vi "WinBuilder._2vi.vi"(6 "nSampleNeeded":i32, 7 "TimeStampNeeded":ext, 8 "Error In":errorcluster, 10 "Wvfrm_ref":T2={"t0"=timestamp(0 s since 1904-01-01), "dt"=1.0, "attributes"=variant, "Y_ref"=refnum} {"dt" format="%0.6f"; "t0" format="%<%X\n%x>T"}, 11 "Fitter In":refnum<class "FitterBase.lvclass">) -> (0 "Error Out":errorcluster, 1 "Valid":bool, 2 "Window":T1={"Timestamp"=0.0, "Samples"=[], "Window Valid"=FALSE, "T0"=-1.0} {"T0" format="%.6f"; "Timestamp" format="%.6f"}, 3 "Fitter Out":refnum<class "FitterBase.lvclass">, 4 "Continue":bool)   [LabVIEW 2018, in "AnalysisPlugins.lvlib" / "FitterBase.lvclass"]
uses:
  FitterBase.lvclass
  Typedefs/clAnalysisConfig.ctl
  Digitizer/DigitizerPlugins/DigitizerBaseClass/Typedefs/WfrmAttributes.ctl
  Digitizer/DigitizerPlugins/DigitizerBaseClass/DigitizerBase.lvclass
  Typedefs/Wvfrm_ref.ctl
  AnalysisPluginBaseClass/Typedefs/clWindowData.ctl
  AnalysisPluginBaseClass/AnalysisPluginsBase.lvclass
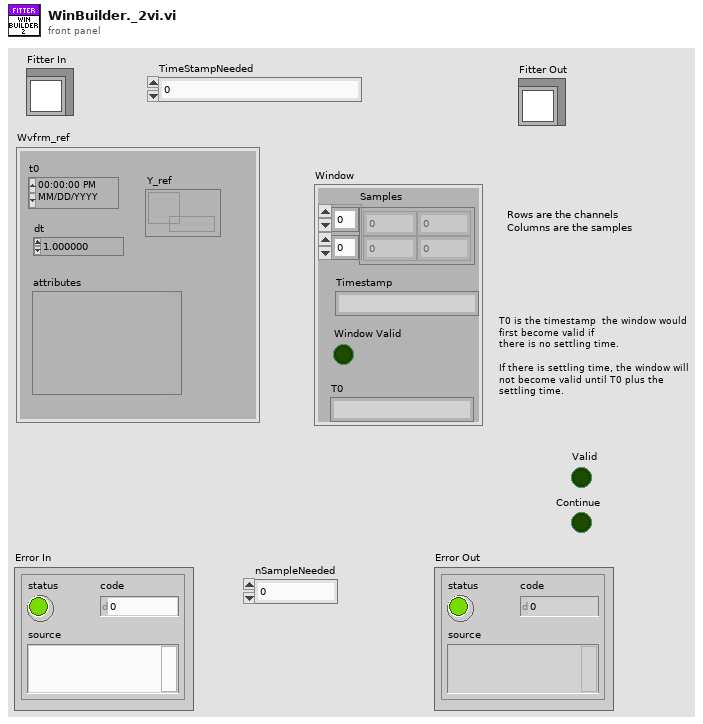
[diagram p1: front panel]
types:
  T1 = typedef "AnalysisPlugins.lvlib/AnalysisPluginsBase.lvclass/clWindowData.ctl" = cluster{"Timestamp":ext, "Samples":dbl[][], "Window Valid":bool, "T0":ext}
  T2 = typedef "AnalysisPlugins.lvlib/FitterBase.lvclass/Wvfrm_ref.ctl" = cluster{"t0":timestamp, "dt":dbl, "attributes":variant, "Y_ref":refnum<data-value>}
  T3 = typedef "DigitizerPlugins.lvlib/DigitizerBase.lvclass/WfrmAttributes.ctl" = cluster{"XOffset":dbl, "ActualPts":i64, "FirstValid":i64}
  T4 = typedef "AnalysisPlugins.lvlib/FitterBase.lvclass/clAnalysisConfig.ctl" = cluster{"F0":u32, "SettlingTime":dbl, "AnalysisCycles":dbl, "SampleRate":dbl, "NumChannels":u32, "TsOffset":enum16{"start", "middle", "end"}}
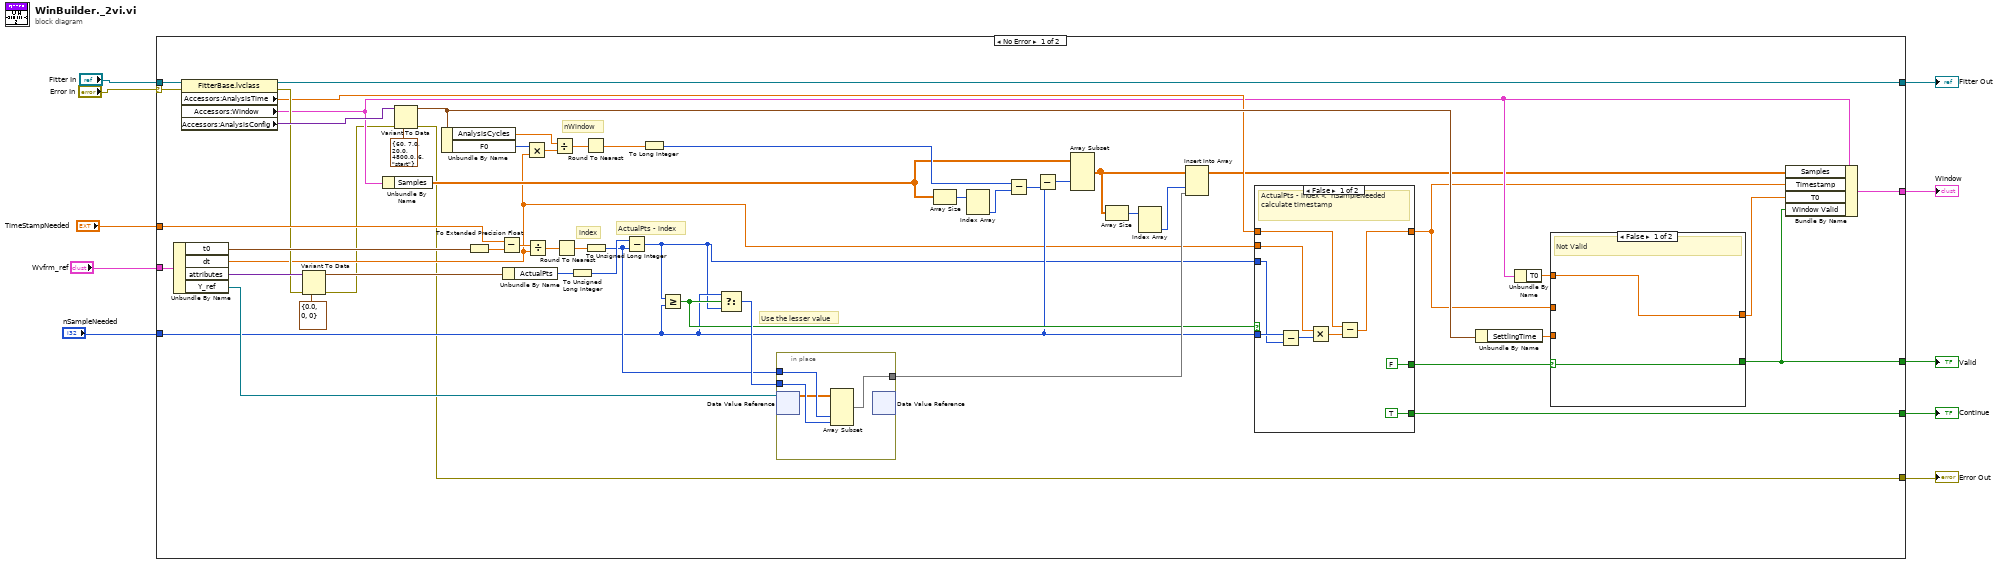
[diagram p0: block diagram]
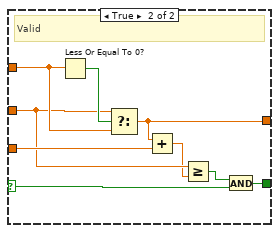
[diagram p2: hidden frame]
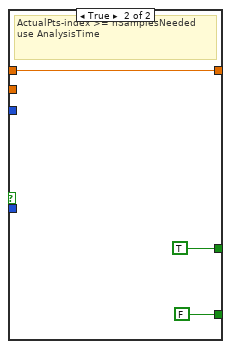
[diagram p3: hidden frame]
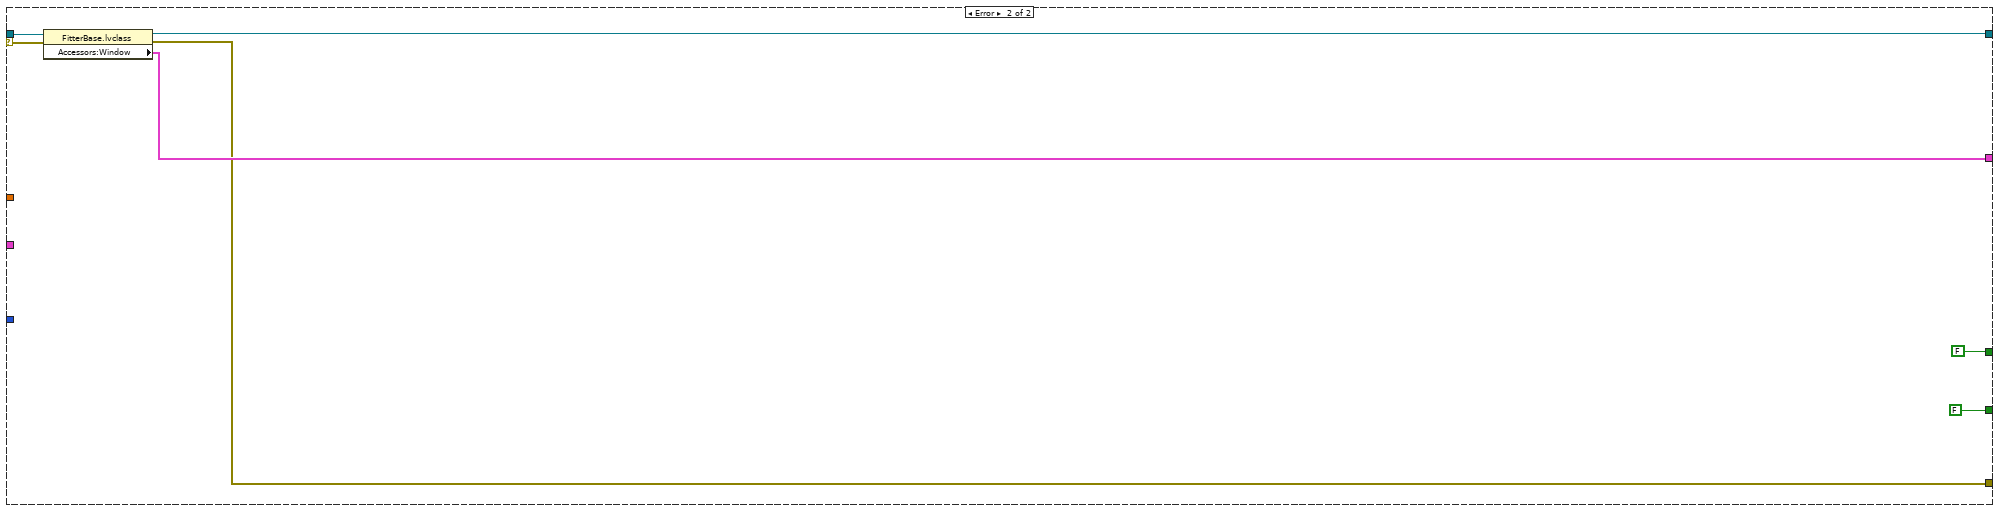
[diagram p4: hidden frame]
diagram:
  n1 = case shown="No Error" "Error In" {
    selector: "Error In" -> [w63 w97]
    tunnel: "Fitter In" -> [w64 w98]
    tunnel: "Wvfrm_ref" -> [w60 _]
    tunnel: "TimeStampNeeded" -> [w57 _]
    tunnel: "nSampleNeeded" -> [w27 _]
    tunnel: [w23 FALSE] -> w5
    tunnel: [w15 FALSE] -> w4
    tunnel: [w14 w94] -> w3
    tunnel: [w13 w93] -> w2
    tunnel: [w11 w92] -> w1
    frame No Error {
      # "nWindow"
      # "Use the lesser value"
      # "ActualPts - index"
      # "index"
      n2 = Unbundle By Name(w60) -> ("t0"=w59:timestamp, "dt"=w25:dbl, "attributes"=w54:variant, "Y_ref"=w47:refnum<data-value>)
      n3 = property class="FitterBase.lvclass"(reference=w64, error in=w63) -> (reference out=w13:refnum<class "FitterBase.lvclass">, error out=w52:errorcluster, "Accessors:AnalysisTime"=w24:dbl, "Accessors:Window"=w22:T1, "Accessors:AnalysisConfig"=w62:variant)
      n4 = Variant To Data(error in=w52, type=T3 {"XOffset"=0.0, "ActualPts"=0, "FirstValid"=0} ("Attributes"), Variant=w54) -> (data=w51:T3, error out=w12:errorcluster)
      n5 = Unbundle By Name(w22) -> ("Samples"=w36:dbl[][])
      n6 = Variant To Data(error in=w12, type=T4 {"F0"=60, "SettlingTime"=7.0, "AnalysisCycles"=20.0, "SampleRate"=4800.0, "NumChannels"=6, "TsOffset"=enum."start"} ("clAnalysisConfig"), Variant=w62) -> (data=w43:T4, error out=w11:errorcluster)
      n7 = Unbundle By Name(w43) -> ("AnalysisCycles"=w40:dbl, "F0"=w42:u32)
      n8 = To Extended Precision Float(1:w59) -> (0:w58:ext)
      n9 = Subtract(x=w57, y=w58) -> (x-y=w56:ext)
      n10 = Unbundle By Name(w51) -> ("ActualPts"=w49:i64)
      n11 = Multiply(x=w42, y=w25) -> (x*y=w41:dbl)
      n12 = Divide(x=w56, y=w25) -> (x/y=w55:ext)
      n13 = Divide(x=w40, y=w41) -> (x/y=w39:dbl)
      n14 = Round To Nearest(number=w55) -> (nearest integer value=w50:ext)
      n15 = To Unsigned Long Integer(number=w49) -> (unsigned 32bit integer=w48:u32)
      n16 = Round To Nearest(number=w39) -> (nearest integer value=w38:dbl)
      n17 = To Unsigned Long Integer(number=w50) -> (unsigned 32bit integer=w45:u32)
      n18 = Subtract(x=w48, y=w45) -> (x-y=w26:u32)
      n19 = To Long Integer(number=w38) -> (32bit integer=w37:i32)
      n20 = Greater Or Equal?(x=w26, y=w27) -> (x >= y?=w28:bool)
      n21 = Select(t=w27, s=w28, f=w26) -> (s? t:f=w46:u32)
      n22 = in-place {
        in-place-border: w45 -> [w89]
        in-place-border: w46 -> [w90]
        in-place-border: [w91] -> w29
        n23 = in-place-dvr #1(w47) -> (w88:dbl[][])  [unwired: 1 out]
        n24 = Array Subset(array=w88, index (col)=w89, length (col)=w90) -> (w91:dbl[][])  [unwired: 2 in]
        n25 = in-place-dvr #1() -> ()  [unwired: 1 in, 2 out]
      }
      n26 = Array Size(array=w36) -> (size(s)=w44:i32[])
      n27 = Index Array(array=w44) -> (element #2=w33:i32)  [unwired: 2 in, 1 out]
      n28 = Subtract(x=w37, y=w33) -> (x-y=w35:i32)
      n29 = Subtract(x=w27, y=w35) -> (x-y=w34:i32)
      n30 = Array Subset(array=w36, index (col)=w34) -> (w31:dbl[][])  [unwired: 3 in]
      n31 = Array Size(array=w31) -> (size(s)=w32:i32[])
      n32 = Index Array(array=w32) -> (element #2=w30:i32)  [unwired: 2 in, 1 out]
      n33 = Insert Into Array(array=w31, index (col)=w30, new element=w29) -> (w21:dbl[][])  [unwired: 1 in]
      n34 = case shown="False" w28 {
        tunnel: [w78 w87] -> w17
        tunnel: w27 -> [w84 _]
        tunnel: w26 -> [w83 _]
        tunnel: w25 -> [w82 _]
        tunnel: w24 -> [w79 w87]
        tunnel: [TRUE FALSE] -> w23
        tunnel: [FALSE TRUE] -> w20
        frame False {
          # "ActualPts - index <  nSampleNeeded\ncalculate timestamp"
          n35 = Subtract(x=w84, y=w83) -> (x-y=w81:u32)
          n36 = Multiply(x=w82, y=w81) -> (x*y=w80:dbl)
          n37 = Subtract(x=w79, y=w80) -> (x-y=w78:dbl)
        }
        frame True {
          # "ActualPts-index >= nSamplesNeeded\nuse AnalysisTime"
        }
      }
      n38 = Unbundle By Name(w43) -> ("SettlingTime"=w18:dbl)
      n39 = Unbundle By Name(w22) -> ("T0"=w19:ext)
      n40 = case shown="False" w20 {
        selector: w20 -> [w65 w69]
        tunnel: w19 -> [w66 w74]
        tunnel: w18 -> [_ w73]
        tunnel: w17 -> [_ w72]
        tunnel: [w65 w68] -> w15
        tunnel: [w66 w67] -> w16
        frame False {
          # "Not Valid"
        }
        frame True {
          # "Valid"
          n41 = Less Or Equal To 0?(x=w74) -> (x <= 0?=w75:bool)
          n42 = Select(t=w72, s=w75, f=w74) -> (s? t:f=w67:ext)
          n43 = Add(x=w67, y=w73) -> (x+y=w71:ext)
          n44 = Greater Or Equal?(x=w72, y=w71) -> (x >= y?=w70:bool)
          n45 = And(x=w70, y=w69) -> (x .and. y?=w68:bool)
        }
      }
      n46 = Bundle By Name(cluster=w22, "Samples"=w21, "Timestamp"=w17, "T0"=w16, "Window Valid"=w15) -> (w14:T1)
    }
    frame Error {
      n47 = property class="FitterBase.lvclass"(reference=w98, error in=w97) -> (reference out=w93:refnum<class "FitterBase.lvclass">, error out=w92:errorcluster, "Accessors:Window"=w94:T1)
    }
  }
  "Fitter Out" <- w2
  "Error Out" <- w1
  "Continue" <- w5
  "Valid" <- w4
  "Window" <- w3
